vi "Untitled 1.vi"() -> ()   [LabVIEW 2020]
panel:
  in  "VISA resource name":refnum<visa-resource-name>
  in  "Table Control":string[][](table)
  out "Waveform Chart  humidity":dbl(graph)
  out "Waveform Chart temp":dbl(graph)
  out "humidity":dbl(knob) scale=0.0..100.0
  out "temperature":dbl(slide) scale=0.0..100.0
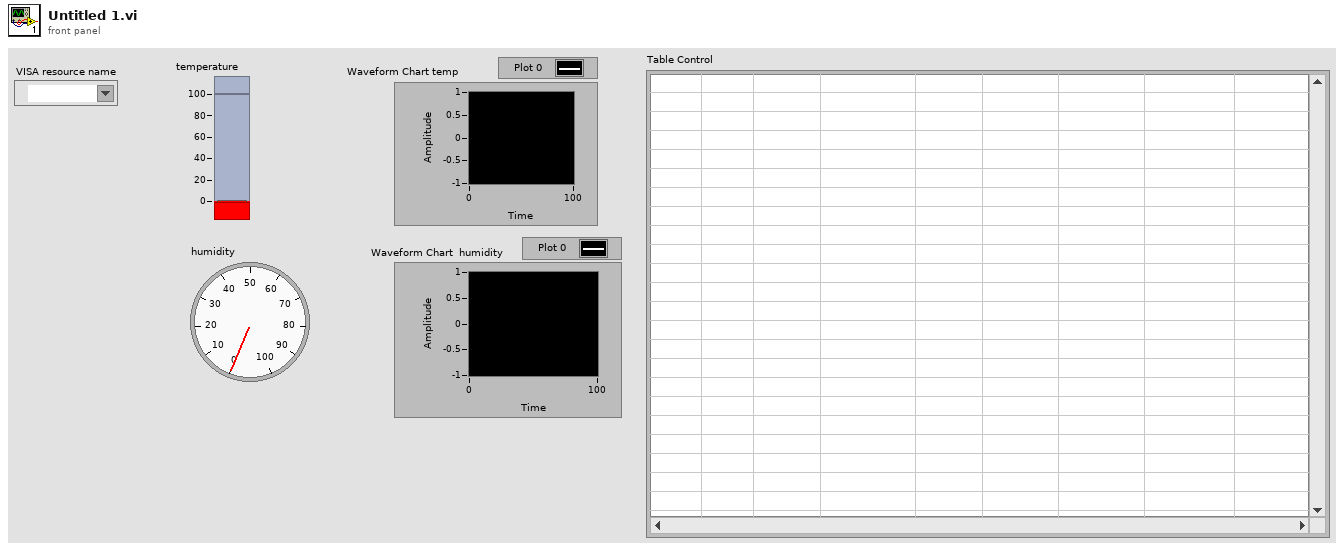
[diagram p1: front panel]
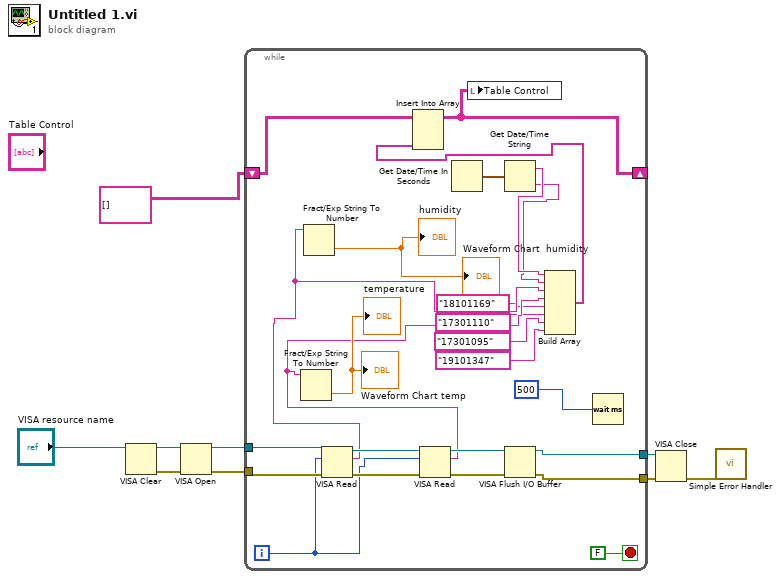
[diagram p0: block diagram]
diagram:
  n1 = VISA Clear(VISA resource name="VISA resource name") -> (VISA resource name out=w9:refnum<visa-resource-name>, error out=w8:errorcluster)  [unwired: 1 in]
  n2 = VISA Open(error in (no error)=w8, VISA resource name=w9) -> (VISA resource name=w7:refnum<visa-resource-name>, error out=w6:errorcluster)  [unwired: 3 in]
  n3 = while {
    tunnel: w7 -> [w34]
    tunnel: w6 -> [w33]
    tunnel: [w28] -> w5
    tunnel: [w27] -> w4
    shift-right: [w23] -> _
    shift-left: string[][] [] -> [w24]
    i -> [w26]
    stop <- FALSE stop-if-true
    n4 = VISA Read(VISA resource name=w34, byte count=w26, error in (no error)=w33) -> (VISA resource name out=w32:refnum<visa-resource-name>, read buffer=w18:string, error out=w31:errorcluster)  [unwired: 1 out]
    n5 = Fract/Exp String To Number(string=w18) -> (number=→"humidity" →"Waveform Chart  humidity":dbl)  [unwired: 3 in, 1 out]
    n6 = VISA Read(VISA resource name=w32, byte count=w26, error in (no error)=w31) -> (VISA resource name out=w30:refnum<visa-resource-name>, read buffer=w17:string, error out=w29:errorcluster)  [unwired: 1 out]
    n7 = Fract/Exp String To Number(string=w17) -> (number=→"temperature" →"Waveform Chart temp":dbl)  [unwired: 3 in, 1 out]
    n8 = Get Date/Time In Seconds() -> (seconds since 1Jan1904=w20:timestamp)
    n9 = Get Date/Time String(seconds (now)=w20) -> (date string=w19:string, time string=w13:string)  [unwired: 2 in]
    n10 = VISA Flush I/O Buffer(VISA resource name=w30, error in (no error)=w29) -> (VISA resource name out=w28:refnum<visa-resource-name>, error out=w27:errorcluster)  [unwired: 1 in]
    n11 = Build Array(w19, w13, w18, w17, "18101169" ("element"), "17301110" ("element"), "17301095" ("element"), "19101347" ("element")) -> (w15:string[])
    n12 = Insert Into Array(array=w24, new element=w15) -> (w23:string[][])  [unwired: 2 in]
    n13 = local write "Table Control"(w23) -> ()
    n14 = Wait (ms)(milliseconds to wait=u32 500) -> ()  [unwired: 1 out]
  }
  n15 = VISA Close(VISA resource name=w5, error in (no error)=w4) -> (error out=w3:errorcluster)
  n16 = call <vilib>:"Simple Error Handler.vi"("error in (no error)"=w3) -> ()  [unwired: 4 in, 5 out]
